vi "Dictionary.Split into DBL and String.vi"(8 "error in (no error)":errorcluster, 11 "Data (Dictionary)":T1[](array[typedef])) -> (0 "error out":errorcluster, 2 "Data (Dictionary) (String)":T1[](array[typedef]), 3 "Data (Dictionary) (Dbl)":T1[](array[typedef]))   [LabVIEW 2016]
uses:
  Data/Typedefs/Dictionary--cluster.ctl
  <vilib>/Utility/Data Type/NI_Data Type.lvlib
  Data/Data.lvclass
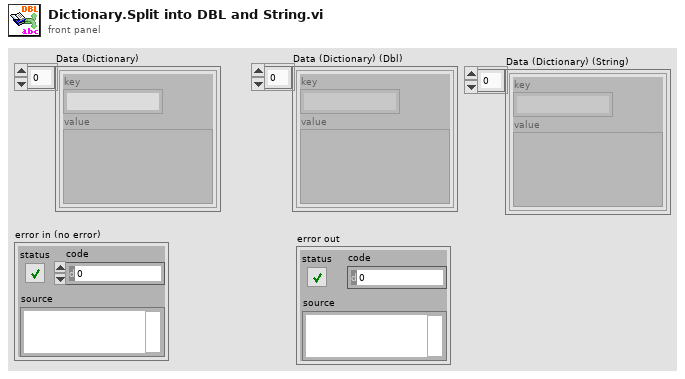
[diagram p1: front panel]
types:
  T1 = typedef "Data.lvclass/Dictionary--cluster.ctl" = cluster{"key":string, "value":variant}
  T2 = typedef "NI_Data Type.lvlib/Data Type.ctl" = enum8{"Invalid Type", "Void", "I8", "I16", "I32", "I64", "U8", "U16", "U32", "U64", "Single Float", "Double Float", "Extended Float", "Single Complex", "Double Complex", "Extended Complex", "Enum U8", "Enum U16", "Enum U32", "Enum U64", "Single Float With Unit", "Double Float With Unit", "Extended Float With Unit", "Single Complex with Unit", "Double Complex with Unit", "Extended Complex with Unit", "Boolean", "String", "Path", "Picture", "Tag", "Array", "Cluster", "Variant", "LV Variant", "Waveform", "Timestamp", "Digital Waveform", "Digital Data", "ExpressData", "Refnum", "External Data", "VI", "Poly VI", "LabVIEW Class Instance", "Fixed Point"}
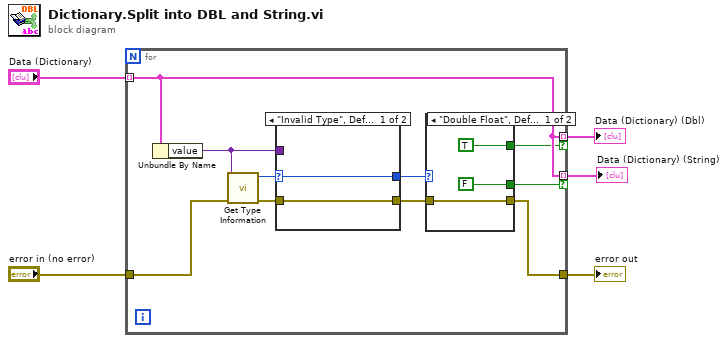
[diagram p0: block diagram]
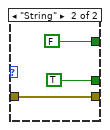
[diagram p2: hidden frame]
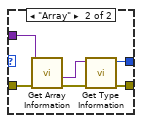
[diagram p3: hidden frame]
diagram:
  n1 = for {
    tunnel: "Data (Dictionary)" -> [w10] mode=indexing
    tunnel: [w10] -> w3 mode=indexing if=w8
    tunnel: [w7] -> w5
    tunnel: "error in (no error)" -> [w15]
    tunnel: [w10] -> w1 mode=indexing if=w9
    n2 = Unbundle By Name(w10) -> ("value"=w12:variant)
    n3 = call <vilib>:"Get Type Information.vi"("error in (no error)"=w15, "Variant"=w12) -> ("error out"=w13:errorcluster, "Type"=w14:T2)  [unwired: 5 in, 3 out]
    n4 = case shown="\"Invalid Type\", Default" w14 {
      selector: w14 -> [w23 _]
      tunnel: w13 -> [w22 w29]
      tunnel: w12 -> [_ w28]
      tunnel: [w22 w25] -> w6
      tunnel: [w23 w24] -> w11
      frame "Invalid Type", Default {
      }
      frame "Array" {
        n5 = call <vilib>:"Get Array Information.vi"("error in (no error)"=w29, "Variant"=w28) -> ("error out"=w27:errorcluster, "Array Element Data Type"=w26:variant)  [unwired: 6 in, 2 out]
        n6 = call <vilib>:"Get Type Information.vi"("error in (no error)"=w27, "Variant"=w26) -> ("error out"=w25:errorcluster, "Type"=w24:T2)  [unwired: 5 in, 3 out]
      }
    }
    n7 = case shown="\"Double Float\", Default" w11 {
      tunnel: [FALSE TRUE] -> w9
      tunnel: [TRUE FALSE] -> w8
      tunnel: [w18 w19] -> w7
      tunnel: w6 -> [w18 w19]
      frame "Double Float", Default {
      }
      frame "String" {
      }
    }
  }
  "error out" <- w5
  "Data (Dictionary) (Dbl)" <- w3
  "Data (Dictionary) (String)" <- w1
